vi "OPC_Step_Selector.vi"(3 "Test Name":string(combo)="DL", 5 "Lane Number":string(combo)="Lane 1") -> (0 "Stork Down":u16, 1 "Stork Up":u16, 2 "Step Force":u16)   [LabVIEW 2017]
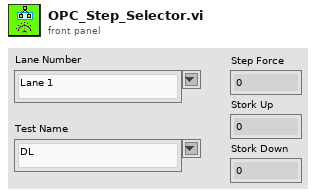
[diagram p1: front panel]
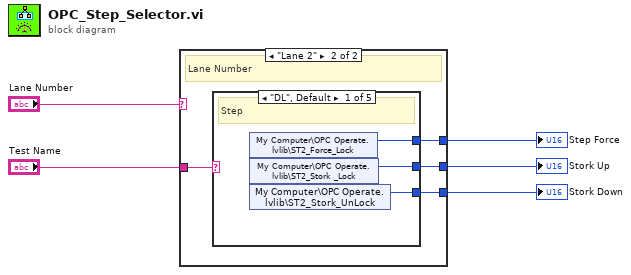
[diagram p0: block diagram]
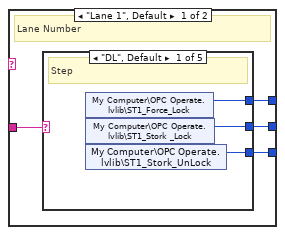
[diagram p2: hidden frame]
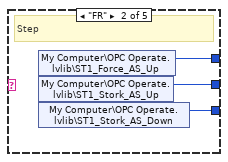
[diagram p3: hidden frame]
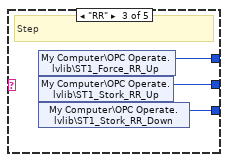
[diagram p4: hidden frame]
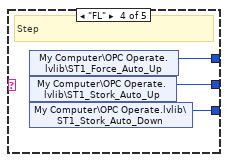
[diagram p5: hidden frame]
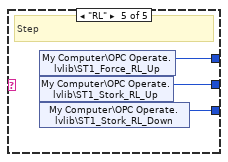
[diagram p6: hidden frame]
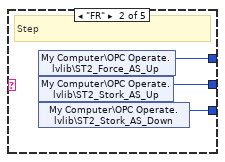
[diagram p7: hidden frame]
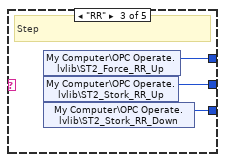
[diagram p8: hidden frame]
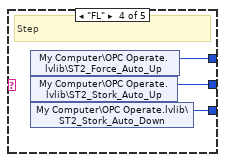
[diagram p9: hidden frame]
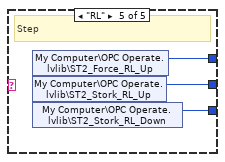
[diagram p10: hidden frame]
diagram:
  n1 = case shown="\"Lane 2\"" "Lane Number" {
    tunnel: "Test Name" -> [w9 w28]
    tunnel: [w8 w27] -> w3
    tunnel: [w7 w26] -> w2
    tunnel: [w6 w25] -> w1
    frame "Lane 1", Default {
      # "Lane Number"
      n2 = case shown="\"DL\", Default" w9 {
        tunnel: [w12 w15 w18 w21 w24] -> w8
        tunnel: [w11 w14 w17 w20 w23] -> w7
        tunnel: [w10 w13 w16 w19 w22] -> w6
        frame "DL", Default {
          # "Step"
          n3 = shared-variable "My Computer\\OPC Operate.lvlib\\ST1_Force_Lock"() -> (w12:u16)  [unwired: 1 in, 1 out]
          n4 = shared-variable "My Computer\\OPC Operate.lvlib\\ST1_Stork _Lock"() -> (w11:u16)  [unwired: 1 in, 1 out]
          n5 = shared-variable "My Computer\\OPC Operate.lvlib\\ST1_Stork_UnLock"() -> (w10:u16)  [unwired: 1 in, 1 out]
        }
        frame "FR" {
          # "Step"
          n6 = shared-variable "My Computer\\OPC Operate.lvlib\\ST1_Force_AS_Up"() -> (w15:u16)  [unwired: 1 in, 1 out]
          n7 = shared-variable "My Computer\\OPC Operate.lvlib\\ST1_Stork_AS_Up"() -> (w14:u16)  [unwired: 1 in, 1 out]
          n8 = shared-variable "My Computer\\OPC Operate.lvlib\\ST1_Stork_AS_Down"() -> (w13:u16)  [unwired: 1 in, 1 out]
        }
        frame "RR" {
          # "Step"
          n9 = shared-variable "My Computer\\OPC Operate.lvlib\\ST1_Force_RR_Up"() -> (w18:u16)  [unwired: 1 in, 1 out]
          n10 = shared-variable "My Computer\\OPC Operate.lvlib\\ST1_Stork_RR_Up"() -> (w17:u16)  [unwired: 1 in, 1 out]
          n11 = shared-variable "My Computer\\OPC Operate.lvlib\\ST1_Stork_RR_Down"() -> (w16:u16)  [unwired: 1 in, 1 out]
        }
        frame "FL" {
          # "Step"
          n12 = shared-variable "My Computer\\OPC Operate.lvlib\\ST1_Force_Auto_Up"() -> (w21:u16)  [unwired: 1 in, 1 out]
          n13 = shared-variable "My Computer\\OPC Operate.lvlib\\ST1_Stork_Auto_Up"() -> (w20:u16)  [unwired: 1 in, 1 out]
          n14 = shared-variable "My Computer\\OPC Operate.lvlib\\ST1_Stork_Auto_Down"() -> (w19:u16)  [unwired: 1 in, 1 out]
        }
        frame "RL" {
          # "Step"
          n15 = shared-variable "My Computer\\OPC Operate.lvlib\\ST1_Force_RL_Up"() -> (w24:u16)  [unwired: 1 in, 1 out]
          n16 = shared-variable "My Computer\\OPC Operate.lvlib\\ST1_Stork_RL_Up"() -> (w23:u16)  [unwired: 1 in, 1 out]
          n17 = shared-variable "My Computer\\OPC Operate.lvlib\\ST1_Stork_RL_Down"() -> (w22:u16)  [unwired: 1 in, 1 out]
        }
      }
    }
    frame "Lane 2" {
      # "Lane Number"
      n18 = case shown="\"DL\", Default" w28 {
        tunnel: [w31 w34 w37 w40 w43] -> w27
        tunnel: [w30 w33 w36 w39 w42] -> w26
        tunnel: [w29 w32 w35 w38 w41] -> w25
        frame "DL", Default {
          # "Step"
          n19 = shared-variable "My Computer\\OPC Operate.lvlib\\ST2_Force_Lock"() -> (w31:u16)  [unwired: 1 in, 1 out]
          n20 = shared-variable "My Computer\\OPC Operate.lvlib\\ST2_Stork _Lock"() -> (w30:u16)  [unwired: 1 in, 1 out]
          n21 = shared-variable "My Computer\\OPC Operate.lvlib\\ST2_Stork_UnLock"() -> (w29:u16)  [unwired: 1 in, 1 out]
        }
        frame "FR" {
          # "Step"
          n22 = shared-variable "My Computer\\OPC Operate.lvlib\\ST2_Force_AS_Up"() -> (w34:u16)  [unwired: 1 in, 1 out]
          n23 = shared-variable "My Computer\\OPC Operate.lvlib\\ST2_Stork_AS_Up"() -> (w33:u16)  [unwired: 1 in, 1 out]
          n24 = shared-variable "My Computer\\OPC Operate.lvlib\\ST2_Stork_AS_Down"() -> (w32:u16)  [unwired: 1 in, 1 out]
        }
        frame "RR" {
          # "Step"
          n25 = shared-variable "My Computer\\OPC Operate.lvlib\\ST2_Force_RR_Up"() -> (w37:u16)  [unwired: 1 in, 1 out]
          n26 = shared-variable "My Computer\\OPC Operate.lvlib\\ST2_Stork_RR_Up"() -> (w36:u16)  [unwired: 1 in, 1 out]
          n27 = shared-variable "My Computer\\OPC Operate.lvlib\\ST2_Stork_RR_Down"() -> (w35:u16)  [unwired: 1 in, 1 out]
        }
        frame "FL" {
          # "Step"
          n28 = shared-variable "My Computer\\OPC Operate.lvlib\\ST2_Force_Auto_Up"() -> (w40:u16)  [unwired: 1 in, 1 out]
          n29 = shared-variable "My Computer\\OPC Operate.lvlib\\ST2_Stork_Auto_Up"() -> (w39:u16)  [unwired: 1 in, 1 out]
          n30 = shared-variable "My Computer\\OPC Operate.lvlib\\ST2_Stork_Auto_Down"() -> (w38:u16)  [unwired: 1 in, 1 out]
        }
        frame "RL" {
          # "Step"
          n31 = shared-variable "My Computer\\OPC Operate.lvlib\\ST2_Force_RL_Up"() -> (w43:u16)  [unwired: 1 in, 1 out]
          n32 = shared-variable "My Computer\\OPC Operate.lvlib\\ST2_Stork_RL_Up"() -> (w42:u16)  [unwired: 1 in, 1 out]
          n33 = shared-variable "My Computer\\OPC Operate.lvlib\\ST2_Stork_RL_Down"() -> (w41:u16)  [unwired: 1 in, 1 out]
        }
      }
    }
  }
  "Step Force" <- w3
  "Stork Up" <- w2
  "Stork Down" <- w1
